vi "CSDB_Config.write Instance.vi"(2 "ClassID":string, 3 "InstanceName":string, 5 "error in (no error)":errorcluster) -> (19 "error out":errorcluster)   [LabVIEW 2014, in "CSDB_Config.lvlib"]
doc: "Adds a new instance to the existing instances of a class."
uses:
  CSDB_Config.lvlib
  <vilib>/addons/database/Connection.llb/Conn Execute.vi
  <vilib>/addons/database/Recordset.llb/Rec Destroy - Connection.vi
  <vilib>/addons/database/NI_Database_API.lvlib
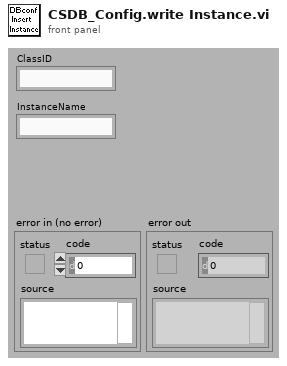
[diagram p1: front panel]
types:
  T1 = typedef "NI_Database_API.lvlib/Conn ObjectReference.ctl" = refnum<k1>
  T2 = typedef "NI_Database_API.lvlib/Rec ObjectReference.ctl" = refnum<k1>
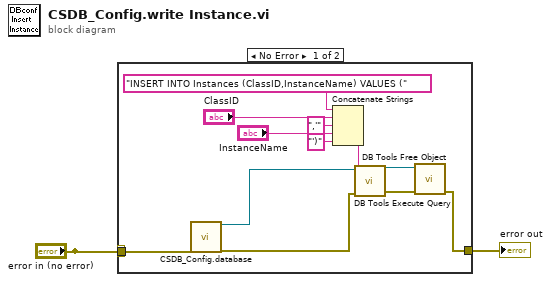
[diagram p0: block diagram]
diagram:
  n1 = case shown="No Error" "error in (no error)" {
    selector: "error in (no error)" -> [_ w15]
    tunnel: "error in (no error)" -> [w8 _]
    tunnel: [w5 w15] -> w2
    frame No Error {
      n2 = call "CSDB_Config.database.vi"("error in (no error)"=w8) -> ("connectionRef out"=w3:T1, "error out"=w4:errorcluster)  [unwired: 17 in]
      n3 = Concatenate Strings("INSERT INTO Instances (ClassID,InstanceName) VALUES (" ("SQL query"), "ClassID", ",'", "InstanceName", "')") -> (w9:string)
      n4 = call-poly <vilib>:"DB Tools Execute Query.vi"("error in (no error)"=w4, "SQL query"=w9, "connection reference"=w3) -> ("error out"=w6:errorcluster, "recordset reference"=w7:T2)  [unwired: 5 in]
      n5 = call-poly <vilib>:"DB Tools Free Object.vi"("error in (no error)"=w6, "recordset reference"=w7) -> ("error out"=w5:errorcluster)  [unwired: 8 in, 1 out]
    }
    frame Error {
    }
  }
  "error out" <- w2
